vi "R-T Fit and Plot_V2.vi"() -> ()   [LabVIEW 2017]
panel:
  out "XY Graph 2":cluster{"T [Celsius]":dbl[], dbl[]}(graph)
  out "Best-Fit Coefficients":dbl[](array[numeric])
  out "XY Graph":T1(graph)
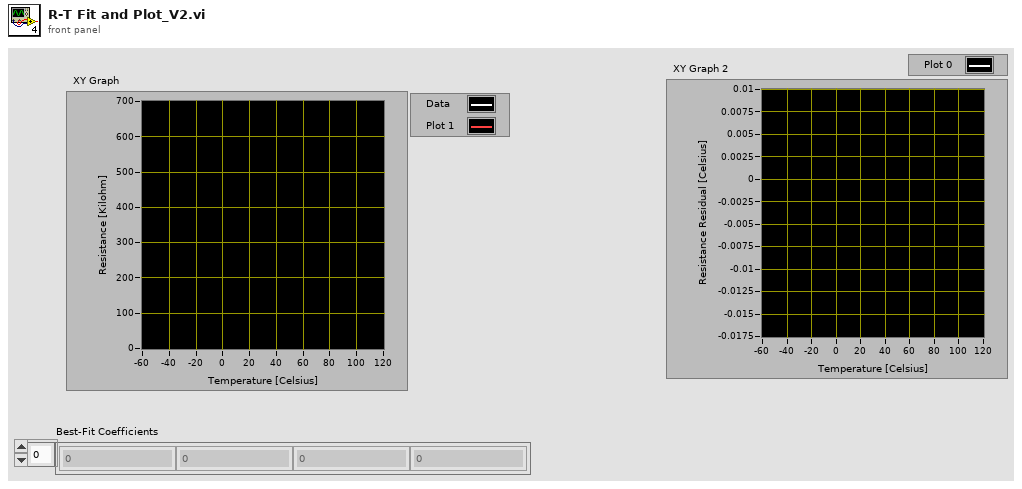
[diagram p1: front panel]
types:
  T1 = cluster{"T [Celsius]":dbl[], "R [kilohm]":dbl[]}[]
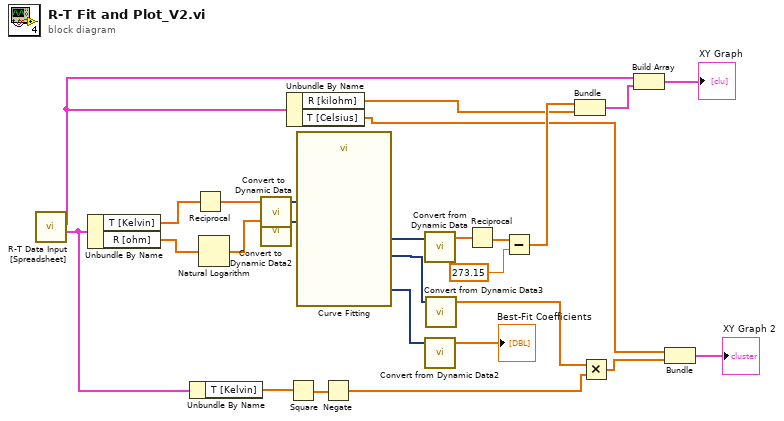
[diagram p0: block diagram]
diagram:
  n1 = call "R-T Data Input [Spreadsheet].vi"() -> ("Kelvin-ohm"=w8:cluster{"T [Kelvin]":dbl[], "R [ohm]":dbl[]}, "Celsius -kilohm"=w10:cluster{"T [Celsius]":dbl[], "R [kilohm]":dbl[]})  [unwired: 10 in]
  n2 = Unbundle By Name(w8) -> ("T [Kelvin]"=w26:dbl[], "R [ohm]"=w25:dbl[])
  n3 = Unbundle By Name(w8) -> ("T [Kelvin]"=w7:dbl[])
  n4 = Reciprocal(x=w26) -> (1/x=w24:dbl[])
  n5 = Natural Logarithm(1:w25) -> (0:w22:dbl[])
  n6 = call "Convert to Dynamic Data"("Array"=w24) -> ("Dynamic Data Type"=w23:dynamicdata)  [unwired: 3 in]
  n7 = call "Convert to Dynamic Data2"("Array"=w22) -> ("Dynamic Data Type"=w21:dynamicdata)  [unwired: 3 in]
  n8 = Unbundle By Name(w10) -> ("R [kilohm]"=w14:dbl[], "T [Celsius]"=w9:dbl[])
  n9 = Square(x=w7) -> (x^2=w6:dbl[])
  n10 = call "Curve Fitting"("Locations"=w21, "Signals"=w23) -> ("residual"=w5:dynamicdata, "best fit"=w20:dynamicdata, "general LS coefficients"=w11:dynamicdata)  [unwired: 5 in, 2 out]
  n11 = Negate(x=w6) -> (-x=w3:dbl[])
  n12 = call "Convert from Dynamic Data"("Dynamic Data Type"=w20) -> ("Array"=w19:dbl[])  [unwired: 3 in]
  n13 = call "Convert from Dynamic Data2"("Dynamic Data Type"=w11) -> ("Array"=→"Best-Fit Coefficients":dbl[])  [unwired: 3 in]
  n14 = call "Convert from Dynamic Data3"("Dynamic Data Type"=w5) -> ("Array"=w4:dbl[])  [unwired: 3 in]
  n15 = Reciprocal(x=w19) -> (1/x=w18:dbl[])
  n16 = Subtract(x=w18, y=273.15) -> (x-y=w15:dbl[])
  n17 = Bundle(w15, "R [kilohm]"=w14) -> (w13:cluster{dbl[], "R [kilohm]":dbl[]})  [unwired: 1 in]
  n18 = Multiply(x=w4, y=w3) -> (x*y=w2:dbl[])
  n19 = Build Array(w10, w13) -> (→"XY Graph":T1)
  n20 = Bundle("T [Celsius]"=w9, w2) -> (→"XY Graph 2":cluster{"T [Celsius]":dbl[], dbl[]})  [unwired: 1 in]
